vi "Pre-Actor.vi"(8 "error in (no error)":errorcluster, 11 "336XX in":refnum<class "336XX.lvclass">) -> (0 "error out":errorcluster, 3 "336XX out":refnum<class "336XX.lvclass">)   [LabVIEW 2019, in "336XX.lvlib" / "336XX.lvclass"]
doc: "This override VI is to provide the means for children classes to perform application specific post launch initialization functions that must be performed *prior* to calling the actor. \n\n***DO NOT USE THE CHECK FOR FAULT ROUTINE HERE***"
uses:
  Library/336XX.lvclass
  C:/Users/Public/Documents/Development/builds/Instruments/FunctionGenerator.lvlibp/Library/FunctionGenerator.lvclass
  builds/Instruments/FunctionGenerator.lvlibp/Accessors/Read NumChans.vi
  builds/Instruments/FunctionGenerator.lvlibp/Library/FunctionGenerator.lvclass
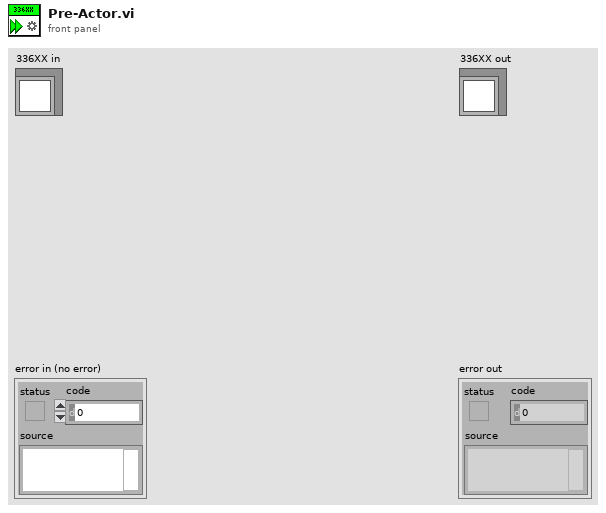
[diagram p1: front panel]
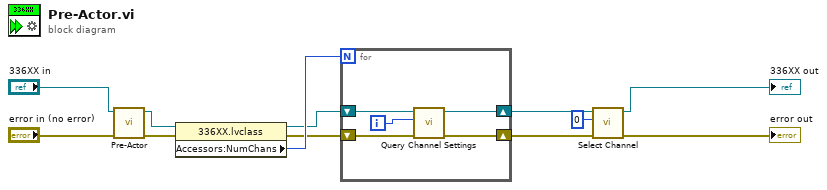
[diagram p0: block diagram]
diagram:
  n1 = call-parent "Pre-Actor.vi"("error in (no error)"="error in (no error)", "FunctionGenerator in"="336XX in") -> ("error out"=w12:errorcluster, "FunctionGenerator out"=w9:refnum<class "336XX.lvclass">)  [unwired: 8 in]
  n2 = property class="336XX.lvclass"(reference=w9, error in=w12) -> (reference out=w7:refnum<class "336XX.lvclass">, error out=w6:errorcluster, "Accessors:NumChans"=w8:i32)
  n3 = for {
    N: w8 -> [_]
    shift-right: [w15] -> w5
    shift-left: w7 -> [w16]
    shift-right: [w14] -> w4
    shift-left: w6 -> [w17]
    i -> [w13]
    n4 = call "Query Channel Settings.vi"("error in (no error)"=w17, "ActiveChannel"=w13, "336XX in"=w16) -> ("error out"=w14:errorcluster, "336XX out"=w15:refnum<class "336XX.lvclass">)  [unwired: 7 in]
  }
  n5 = call "Select Channel.vi"("error in (no error)"=w4, "Active Channel"=0, "FunctionGenerator in"=w5) -> ("error out"=→"error out":errorcluster, "FunctionGenerator out"=→"336XX out":refnum<class "336XX.lvclass">)  [unwired: 7 in]
